vi "Check Database.vi"() -> (3 "Database Check Results":T1)   [LabVIEW 2026, in "Readines Service.lvclass"]
uses:
  Readines Service.lvclass
  Readines Service.lvclass/Readines Service.ctl
  Typedefs/enums/Readiness State Enum.ctl
  Typedefs/clusters/Readiness Check Result.ctl
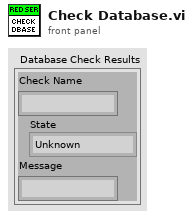
[diagram p1: front panel]
types:
  T1 = typedef "Readiness Check Result.ctl" = cluster{"Check Name":string, "State":T2, "Message":string}
  T2 = typedef "Readiness State Enum.ctl" = enum16{"Unknown", "Ready", "Warning", "NotReady"}
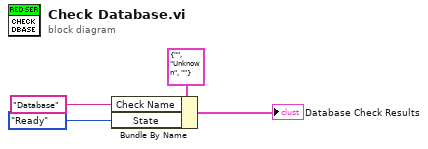
[diagram p0: block diagram]
diagram:
  n1 = Bundle By Name(cluster=T1 {"Check Name"="", "State"=enum."Unknown", "Message"=""} ("Readiness Check Result"), "Check Name"="Database", "State"=Readiness_State_Enum."Ready") -> (→"Database Check Results":T1)
